vi "RunWireCalibration.vi"() -> ()   [LabVIEW 2016]
uses:
  Controls/0_XYZstage/BOOL_Moving.ctl
  <vilib>/userdefined/High Color/IMAQdx.ctl
  <vilib>/Utility/miscctls.llb/LVRowAndColumnUnsignedTypeDef.ctl
  <vilib>/Analysis/6fits.llb/Curve Fitting Criteria.ctl
  <extravilib>/ChannelInstances/High Speed Stream-c(i32,str,c(dbl,dbl),t'IMAQ Image.ctl',t'IMAQdx.ctl')/_Read For Replicate.vi
  Miscellaneous/PixelToMicron.vi
  <extravilib>/ChannelInstances/High Speed Stream-c(i32,str,c(dbl,dbl),t'IMAQ Image.ctl',t'IMAQdx.ctl')/Instantiate.vi
  <extravilib>/ChannelInstances/High Speed Stream-c(i32,str,c(dbl,dbl),t'IMAQ Image.ctl',t'IMAQdx.ctl')/)Channel.vi
  <extravilib>/ChannelInstances/High Speed Stream-c(i32,str,c(dbl,dbl),t'IMAQ Image.ctl',t'IMAQdx.ctl')/Abort Signal/Init Signal.vi
  <vilib>/gmath/statdist.llb/st_Percentiles (scalar).vi
  <vilib>/vision/driver/NI_Vision_Acquisition_Software.lvlib
  <vilib>/Analysis/NI_AALPro.lvlib
  <vilib>/Analysis/NI_AALBase.lvlib
  <vilib>/gmath/NI_Gmath.lvlib
  <vilib>/LabVIEW Interface for Arduino/LabVIEW Interface for Arduino.lvlib
  <extravilib>/ChannelInstances/High Speed Stream-c(i32,str,c(dbl,dbl),t'IMAQ Image.ctl',t'IMAQdx.ctl').lvlib
panel:
  out "completed":bool
  out "Loops":i32
  out "Image Data":T1(array[cluster])
  in  "Mode":enum16{"Run Calibration", "View Results"}(ring)
  out "Finished":bool
  in  "Tab Control":T2(tab)
  in  "error tab":bool
  in  "cam session":T3="cam1" caption="Select Camera"
  in  "Short-distance\naxis speed":T4={"vX [mm/s]"=5.0, "vY [mm/s]"=5.0, "vZ [mm/s]"=5.0}
  in  "Long-distance\naxis speed":T4={"vX [mm/s]"=25.0, "vY [mm/s]"=12.5, "vZ [mm/s]"=5.0}
  in  "wait time":u32=2000 caption="wait (ms)"
  in  "Y position":dbl=86.5 format="%#_13g"
  in  "Z position":dbl=30.25 format="%#_13g"
  in  "percentile":dbl=95.0 caption="tolerance percentile" format="%#_13g"
  in  "Python":path=path "python"
  in  "Wire Diameter":dbl=90.0 caption="Wire Diameter (microns)"
  in  "Image Info Results Read":path caption="Image Info Path"
  in  "Image File Results Read":bool=TRUE caption="View Images from Saved Location?"
  in  "Im. Source":T5(radio)
  out "Image Source Tab":T5(tab) caption="Warning: if you don't save the images, a new set of images must be captured to run the calibration again. Saving images allows the user to run the calibration on the same image set multiple times."
  in  "Save Images":bool=TRUE caption="Save Images to File?"
  in  "Image Calibration Write":path=path "C:/Users/Aerotech/Desktop/Joel Images 8_7" caption="Image Path"
  in  "Image Overwrite":bool=TRUE caption="Overwrite existing files?"
  in  "Image Info Calibration Read":path caption="Image Info Path"
  in  "View Results":bool
  in  "Data File Read":path caption="Data File Path"
  in  "Run Calibration":bool
  in  "File Name":string="data_file.csv"
  in  "Data File Overwrite":bool caption="Overwrite existing files?"
  in  "Data File Write":path=path "C:/Users/Aerotech/Desktop" caption="Data File Path"
  in  "List of All Fits":i32(listbox)
  out "Progress":dbl(slide) caption="Progress: 378/719" scale=0.0..100.0
  out "Moving":T6
  in  "abort":bool
  in  "pause":bool
  out "Graph of Fit":cluster{dbl[], dbl[]}[](graph) caption="Graph of Fit for Image #15"
  in  "List of Failed Fits":i32(listbox)
  out "Image":T7(plugin-control) caption="Image #15"
  out "Fit Info":T8={"Initial Guess"={"Center (pixels)"=-1.0, "Reflectivity"=0.0}, "Params Vector"=[], "Errors"=[], "Iterations"=0, "Success"=FALSE} {"Errors" format="%#_2g"; "Params Vector" format="%#_10f"; "Initial Guess"."Center (pixels)" format="%#_16g"}
  in  "Quit":bool
  out "Re-do Necessary?":bool
  out "fails":i32 caption="Number of Failed Fits:"
  out "Tolerance":dbl=4.0 caption="95% Tolerance (microns):" format="%_2g"
  out "Confidence":dbl caption="95% Confidence Interval (microns):" format="%.5g"
  out "std. dev.":dbl caption="Standard Deviation (microns):" format="%.5g"
  out "outside tolerance":bool caption="Within Tolerance?"
  out "Histogram of Final Fit Residuals":T9(graph) caption="XY Graph"
  out "Adjusted Graph of Final Fit":cluster{dbl[], dbl[]}(graph) caption="XY Graph"
  out "queue error":errorcluster
  out "image file error":errorcluster
  out "info file error":errorcluster
  out "Image Display Error":errorcluster
  out "data file write error":errorcluster
  out "Capture Error":errorcluster caption="stage/camera error"
  # "NOTE: Click \"RUN\" to run the VI BEFORE entering the set-up parameters!!!"
  # "For runnung a new calibration"
  # "For viewing a previously run calibration"
  # "Image Files"
  # "Settings"
  # "Image Files"
  # "Data File"
  # "Data File"
  # "Center (px)"
  # "Reflectivity (ul)"
  # "Amplitude (px val^2)"
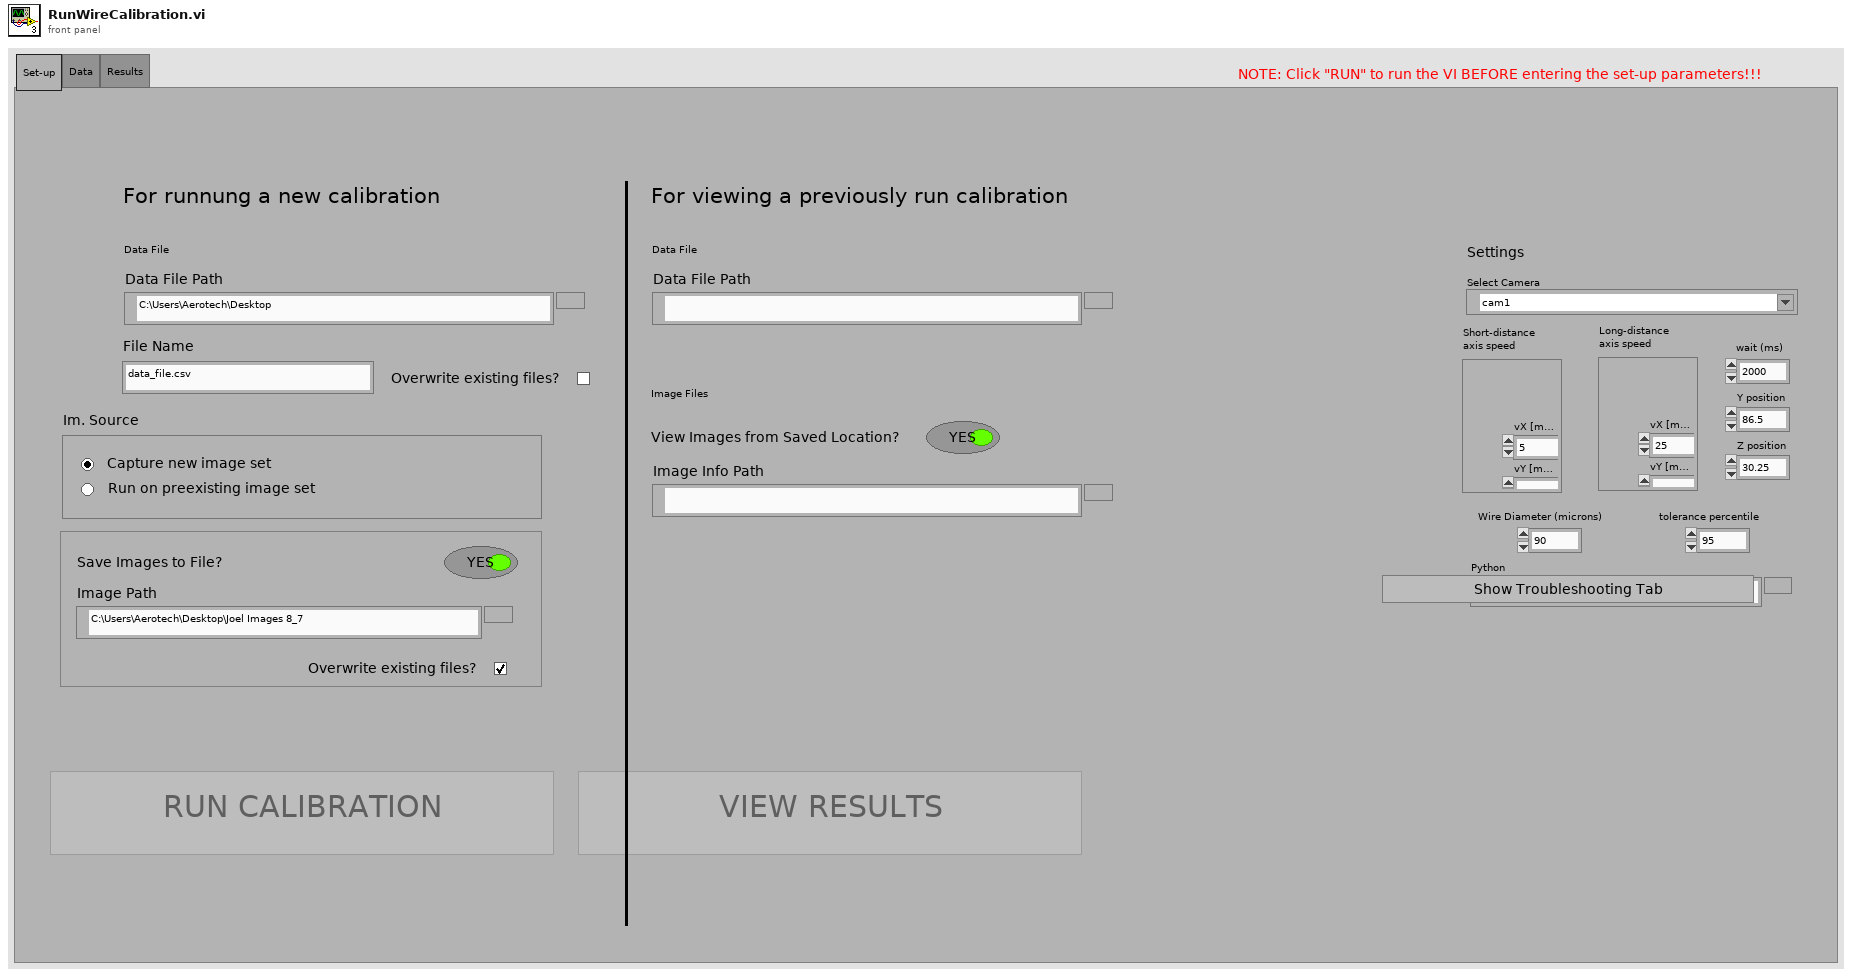
[diagram p1: front panel]
types:
  T1 = cluster{"success?":bool, "image number":i32, "camera position":cluster{"X":dbl, "Y":dbl}, "parameters":cluster{"amplitude":dbl, "center":dbl, "reflectivity":dbl}, "errors":cluster{"amplitude":dbl, "center":dbl, "reflectivity":dbl}, "Initial Guess":cluster{"center":dbl, "reflectivity":dbl}, "iterations":i32, "image path":path}[]
  T2 = enum32{"Set-up", "Data", "Results", "Troubleshooting"}
  T3 = typedef "IMAQdx.ctl" = refnum<k21>
  T4 = cluster{"vX [mm/s]":dbl, "vY [mm/s]":dbl, "vZ [mm/s]":dbl}
  T5 = enum32{"Capture new image set", "Run on preexisting image set"}
  T6 = typedef "BOOL_Moving.ctl" = bool
  T7 = typedef "IMAQ Image.ctl" = refnum<image>
  T8 = cluster{"Initial Guess":cluster{"Center (pixels)":dbl, "Reflectivity":dbl}, "Params Vector":dbl[], "Errors":dbl[], "Iterations":i32, "Success":bool}
  T9 = cluster{"X Values":dbl[], "Histogram: h(x)":i32[]}
  T10 = enum8{"Enabled", "Disabled", "Disabled and Grayed Out"}
  T11 = cluster{"Params Vector[1]":dbl, "Params Vector[2]":dbl}
  T12 = enum16{"open", "replace", "create", "open or create", "replace or create", "replace or create with confirmation"}
  T13 = cluster{"image number":i32, "image path":path, "position":cluster{dbl, dbl}}
  T14 = typedef "LVRowAndColumnUnsignedTypeDef.ctl" = cluster{"Row":u32, "Column":u32}
  T15 = cluster{"Data File Write":path, "File Name":string, "Data File Overwrite":bool}
  T16 = typedef "LabVIEW Interface for Arduino.lvlib/Arduino Resource.ctl" = cluster{"VISA resource":refnum<visa-resource-name>, "Board Type":T17, "Connection Type":enum8{"USB / Serial"}, "Bytes Per Packet (15)":u8}
  T17 = typedef "LabVIEW Interface for Arduino.lvlib/Board Type.ctl" = enum16{"Uno", "Dimuelanove w/Atmega 328", "Mega 2560"}
  T18 = typedef "ArduinoLT-ConfigurationControl.ctl" = cluster{"Lights: Digital I/O Pins":cluster{"Coaxial":u8, "Spotlights":u8}, "Thermistor Settings":cluster{"Analogue Readout Pin":u8, "Vcc Reference Pin":u8, "Paired Resistance (10K Ohms)":dbl, "Units (C)":enum16{"Celsius", "Fahrenheit", "Kelvin"}}}
  T19 = cluster{"Image Calibration Write":path, "Image Overwrite":bool}
  T20 = cluster{"Arduino Configuration OUT":T18, "Arduino Resource OUT":T16, "error out":errorcluster}
  T21 = typedef "Image Type" = u32
  T22 = cluster{"Final X":dbl, "Final Y":dbl, "Final Z":dbl}
  T23 = cluster{i32, string, cluster{"Final X":dbl, "Final Y":dbl}, "Image Out":T7, "Session Out":T3}
  T24 = typedef "High Speed Stream-c(i32,str,c(dbl,dbl),t'IMAQ Image.ctl',t'IMAQdx.ctl').lvlib/)Channel.ctl" = refnum<queue>
  T25 = cluster{i32, "Smart Path":path, cluster{"Final X":dbl, "Final Y":dbl}}
  T26 = cluster{i32, "appended path":path, cluster{dbl, dbl}}
  T27 = cluster{"Params Vector[0]":dbl, "Params Vector[1]":dbl, "Params Vector[2]":dbl}
  T28 = cluster{"Errors[0]":dbl, "Errors[1]":dbl, "Errors[2]":dbl}
  T29 = cluster{"Success":bool, "image number":i32, "position":cluster{dbl, dbl}, "Params Vector":cluster{"Params Vector[0]":dbl, "Params Vector[1]":dbl, "Params Vector[2]":dbl}, "Errors":cluster{"Errors[0]":dbl, "Errors[1]":dbl, "Errors[2]":dbl}, cluster{"Params Vector[1]":dbl, "Params Vector[2]":dbl}, "Iterations":i32, "image path":path}
  T30 = cluster{"Success":bool, "image number":i32, "position":cluster{"X":dbl, "Y":dbl}, "Params Vector":cluster{"Params Vector[0]":dbl, "Params Vector[1]":dbl, "Params Vector[2]":dbl}, "Errors":cluster{"Errors[0]":dbl, "Errors[1]":dbl, "Errors[2]":dbl}, "Initial Guess":cluster{"Params Vector[1]":dbl, "Params Vector[2]":dbl}, "Iterations":i32, "image path":path}[]
  T31 = cluster{bool, i32, cluster{dbl, dbl}, cluster{dbl, dbl, dbl}, cluster{dbl, dbl, dbl}, cluster{dbl, dbl}, i32, "appended path":path}
  T32 = typedef "NI_AALPro.lvlib/Curve Fitting Criteria.ctl" = u16
  T33 = cluster{"success?":bool, "image number":i32, "camera position":cluster{"X":dbl, "Y":dbl}, "parameters":cluster{"amplitude":dbl, "center":dbl, "reflectivity":dbl}, "errors":cluster{"amplitude":dbl, "center":dbl, "reflectivity":dbl}, "Initial Guess":cluster{"center":dbl, "reflectivity":dbl}, "iterations":i32, "image path":path}
  T34 = cluster{"amplitude":dbl, "center":dbl, "reflectivity":dbl}
  T35 = cluster{"Initial Guess":cluster{"center":dbl, "reflectivity":dbl}, "parameters":dbl[], "errors":dbl[], "iterations":i32, "success?":bool}
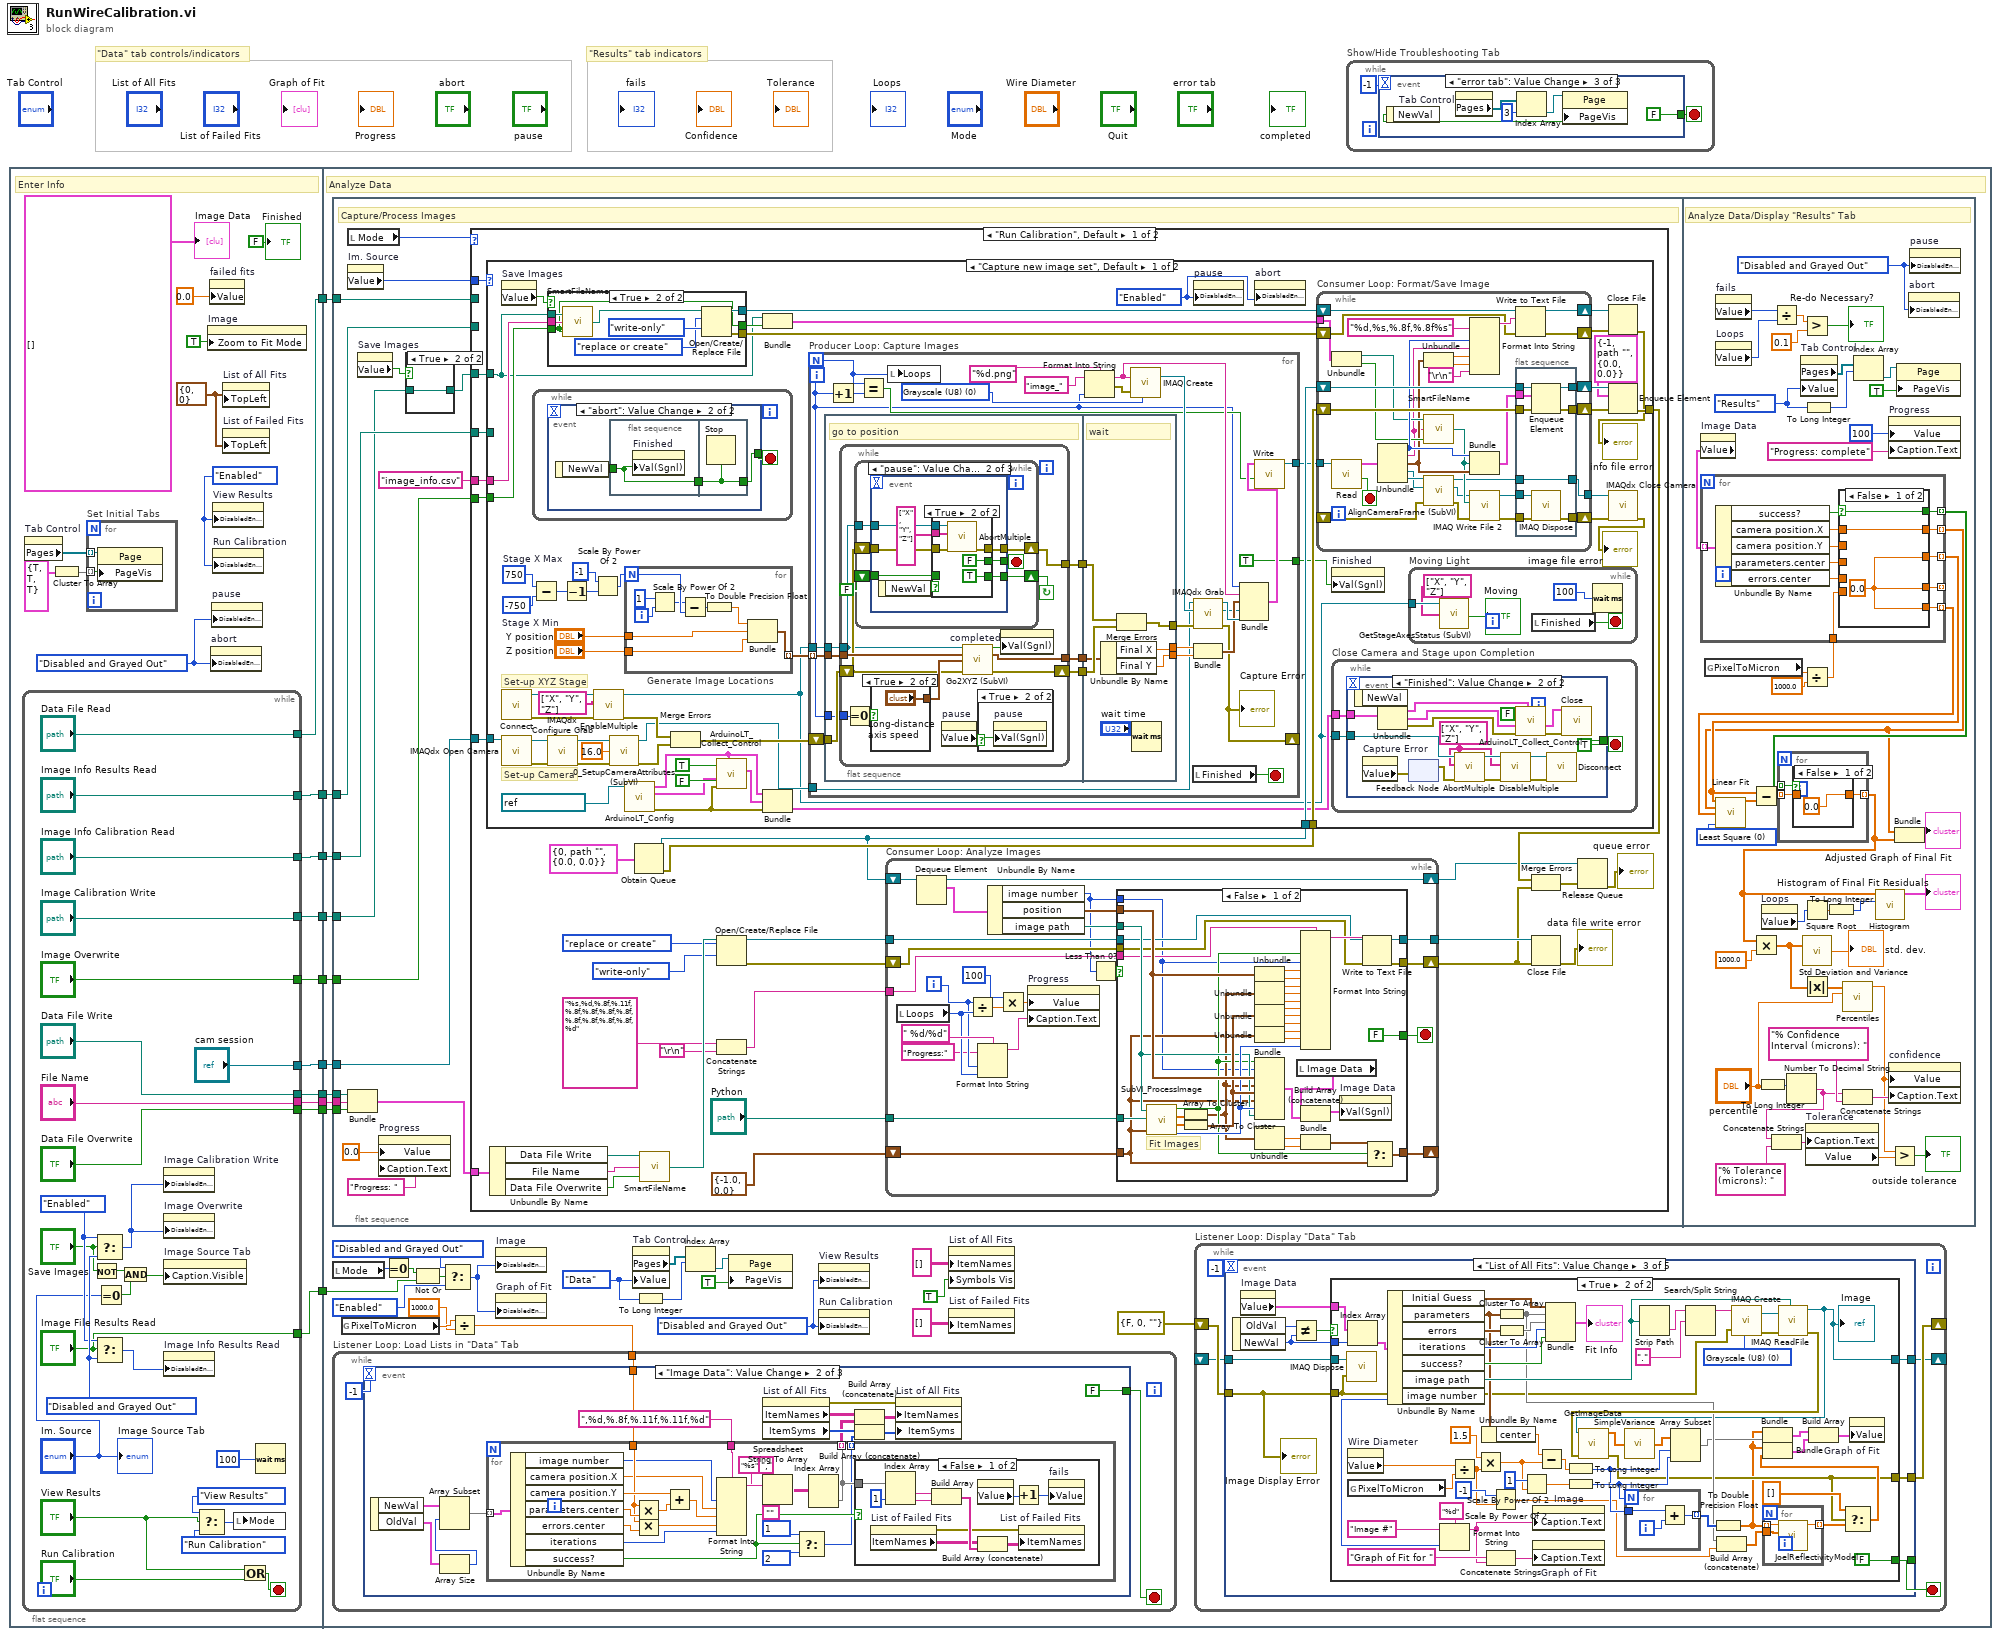
[diagram p0: block diagram]
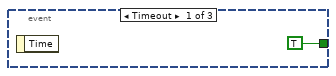
[diagram p2: hidden frame]
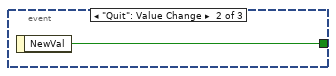
[diagram p3: hidden frame]
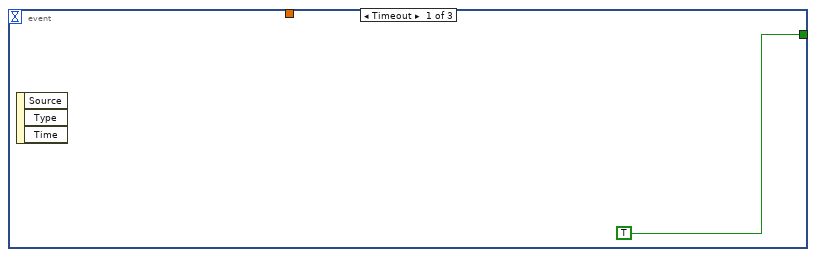
[diagram p4: hidden frame]
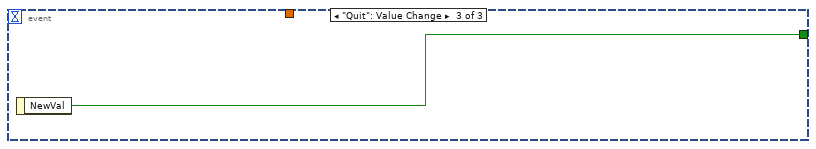
[diagram p6: hidden frame]
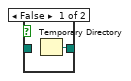
[diagram p7: hidden frame]
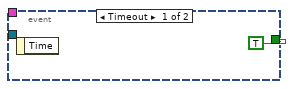
[diagram p8: hidden frame]
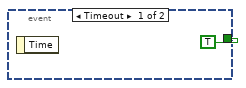
[diagram p9: hidden frame]
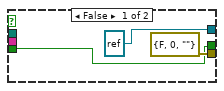
[diagram p10: hidden frame]
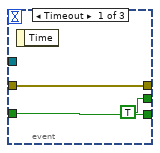
[diagram p12: hidden frame]
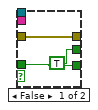
[diagram p13: hidden frame]
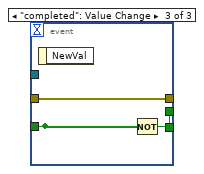
[diagram p14: hidden frame]
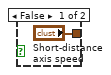
[diagram p15: hidden frame]
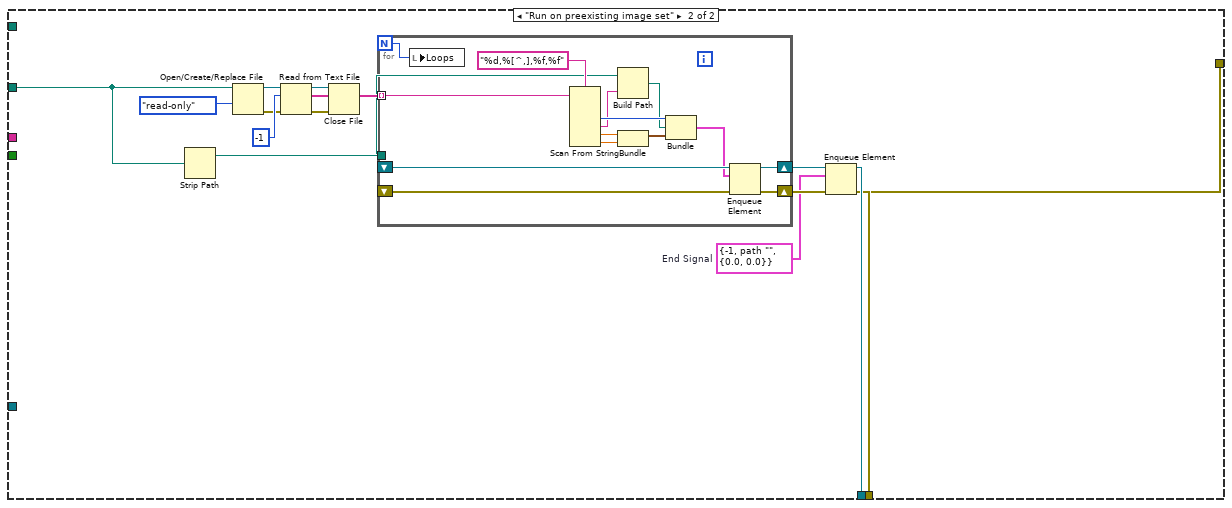
[diagram p16: hidden frame]
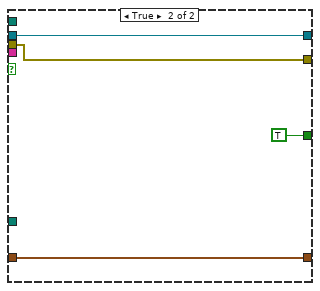
[diagram p17: hidden frame]
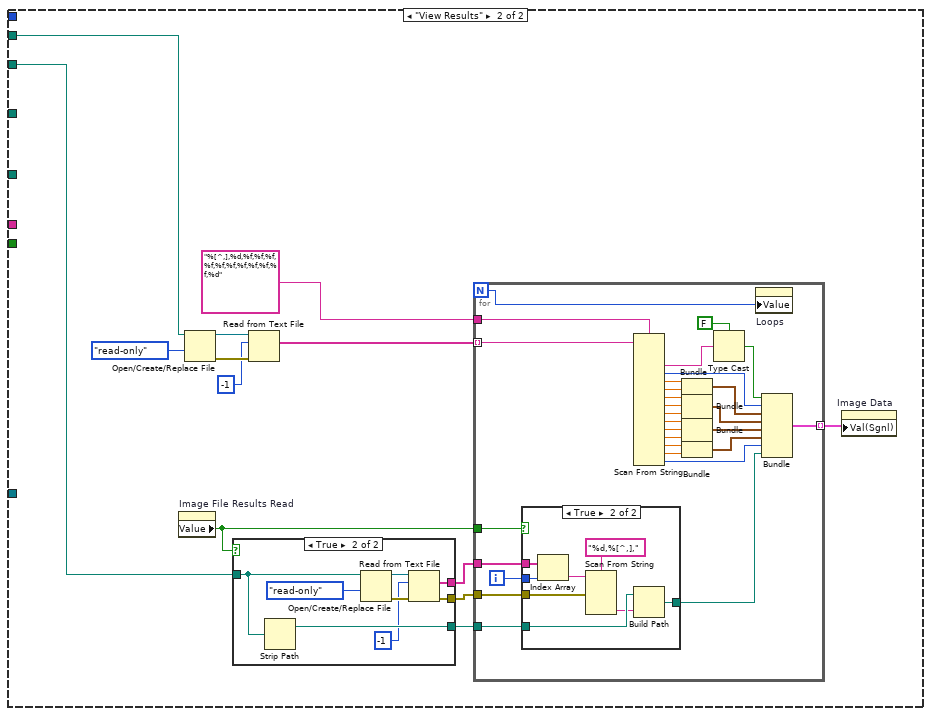
[diagram p18: hidden frame]
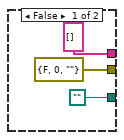
[diagram p19: hidden frame]
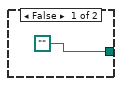
[diagram p20: hidden frame]
diagram:
  # "\"Results\" tab indicators"
  # "\"Data\" tab controls/indicators"
  n1 = flat-sequence {
    tunnel: [w21] -> w10
    tunnel: [w23] -> w9
    tunnel: [w29] -> w8
    tunnel: [w28] -> w7
    tunnel: [w27] -> w6
    tunnel: [w26] -> w5
    tunnel: [w25] -> w4
    tunnel: [w24] -> w3
    tunnel: [w22] -> w2
    tunnel: [w14] -> w1
    tunnel: w10 -> [w79]
    tunnel: w9 -> [w78]
    tunnel: w8 -> [w77]
    tunnel: w7 -> [w72]
    tunnel: w6 -> [w71]
    tunnel: w5 -> [w70]
    tunnel: w4 -> [w69]
    tunnel: w3 -> [w68]
    tunnel: w2 -> [w67]
    tunnel: w1 -> [w60]
    frame #0 {
      w12 = T10."Disabled and Grayed Out" ("Disabled")
      w13 = T10."Enabled" ("Disabled")
      w18 = T14 {"Row"=0, "Column"=0} ("Top Left Visible Cell")
      # "Enter Info"
      n2 = while {
        tunnel: ["Image Overwrite"] -> w29
        tunnel: ["Data File Write"] -> w28
        tunnel: ["File Name"] -> w27
        tunnel: ["Data File Overwrite"] -> w26
        tunnel: ["cam session"] -> w25
        tunnel: ["Image Calibration Write"] -> w24
        tunnel: ["Image Info Calibration Read"] -> w23
        tunnel: ["Image Info Results Read"] -> w22
        tunnel: ["Data File Read"] -> w21
        tunnel: ["Image File Results Read"] -> w14
        stop <- w46 stop-if-true
        w53 = T10."Enabled" ("Disabled")
        w54 = T10."Disabled and Grayed Out" ("Disabled")
        n3 = Not(x="Save Images") -> (.not. x?=w38:bool)
        n4 = Select(t=w53, s="Save Images", f=w54) -> (s? t:f=w52:T10)
        n5 = Select(t=w53, s="Image File Results Read", f=w54) -> (s? t:f=w40:T10)
        n6 = Equal To 0?(x="Im. Source") -> (x = 0?=w36:bool)
        n7 = And(x=w38, y=w36) -> (x .and. y?=w37:bool)
        n8 = property on="Image Calibration Write" class="Path"("DisabledEnum"=w52) -> ()  [unwired: 2 in, 2 out]
        n9 = property on="Image Overwrite" class="Bool (strict)"("DisabledEnum"=w52) -> ()  [unwired: 2 in, 2 out]
        n10 = property on="Image Source Tab" class="TabCtl (strict)"("Caption.Visible"=w37) -> ()  [unwired: 2 in, 2 out]
        n11 = property on="Image Info Results Read" class="Path"("DisabledEnum"=w40) -> ()  [unwired: 2 in, 2 out]
        n12 = Select(t=enum16{"Run Calibration", "View Results"}."View Results" ("Mode"), s="View Results", f=enum16{"Run Calibration", "View Results"}."Run Calibration" ("Mode")) -> (s? t:f=w51:enum16{"Run Calibration", "View Results"})
        n13 = local write "Mode"(w51) -> ()
        n14 = Or(x="View Results", y="Run Calibration") -> (x .or. y?=w46:bool)
        n15 = Wait (ms)(milliseconds to wait=u32 100) -> ()  [unwired: 1 out]
        "Image Source Tab" <- "Im. Source"
      }
      n16 = property on="Tab Control" class="TabCtl (strict)"() -> ("Pages"=w17:refnum<vi>[])  [unwired: 2 in, 2 out]
      n17 = Cluster To Array(cluster=cluster{bool, bool, bool} {TRUE, TRUE, TRUE}) -> (array=w15:bool[])
      n18 = for "Set Initial Tabs" {
        tunnel: w17 -> [w32] mode=indexing
        tunnel: w15 -> [w31] mode=indexing
        n19 = property class="Page"(reference=w32, "PageVis"=w31) -> ()  [unwired: 1 in, 2 out]
      }
      n20 = property on="Image" class="ImageControl"("Zoom to Fit Mode"=TRUE) -> ()  [unwired: 2 in, 2 out]
      n21 = property on="failed fits" class="DigNum (strict)"("Value"=0.0 ("Number of Failed Fits:")) -> ()  [unwired: 2 in, 2 out]
      n22 = property on="abort" class="Bool"("DisabledEnum"=w12) -> ()  [unwired: 2 in, 2 out]
      n23 = property on="pause" class="Bool (strict)"("DisabledEnum"=w12) -> ()  [unwired: 2 in, 2 out]
      n24 = property on="View Results" class="Bool"("DisabledEnum"=w13) -> ()  [unwired: 2 in, 2 out]
      n25 = property on="Run Calibration" class="Bool"("DisabledEnum"=w13) -> ()  [unwired: 2 in, 2 out]
      n26 = property on="List of All Fits" class="MCListbox (strict)"("TopLeft"=w18) -> ()  [unwired: 2 in, 2 out]
      n27 = property on="List of Failed Fits" class="MCListbox (strict)"("TopLeft"=w18) -> ()  [unwired: 2 in, 2 out]
      "Image Data" <- T1 []
      "Finished" <- FALSE ("Finished")
    }
    frame #1 {
      w59 = T10."Disabled and Grayed Out" ("Disabled")
      w81 = T2."Data" ("Tab Control")
      # "Analyze Data"
      n28 = flat-sequence {
        tunnel: w79 -> [w153]
        tunnel: w78 -> [w142]
        tunnel: w77 -> [w152]
        tunnel: w72 -> [w150]
        tunnel: w71 -> [w149]
        tunnel: w70 -> [w148]
        tunnel: w69 -> [w146]
        tunnel: w68 -> [w140]
        tunnel: w67 -> [w145]
        frame #0 {
          # "Capture/Process Images"
          n29 = local read "Mode"() -> (w155:enum16{"Run Calibration", "View Results"})
          n30 = property on="Im. Source" class="RadioBtnsControl (strict)"() -> ("Value"=w154:T5)  [unwired: 2 in, 2 out]
          n31 = Bundle("Data File Write"=w150, "File Name"=w149, "Data File Overwrite"=w148) -> (w147:T15)  [unwired: 1 in]
          n32 = property on="Save Images" class="Bool (strict)"() -> ("Value"=w139:bool)  [unwired: 2 in, 2 out]
          n33 = property on="Progress" class="Slide (strict)"("Value"=0.0 ("Progress"), "Caption.Text"="Progress: ") -> ()  [unwired: 2 in, 2 out]
          n34 = case shown="True" w139 {
            tunnel: [w156 w157] -> w141
            tunnel: w140 -> [_ w157]
            frame False {
              n35 = Temporary Directory() -> (w156:path)
            }
            frame True {
            }
          }
          n36 = case shown="\"Run Calibration\", Default" w155 {
            tunnel: w154 -> [w186 _]
            tunnel: w147 -> [w180 _]
            tunnel: w153 -> [_ w529]
            tunnel: w145 -> [_ w523]
            tunnel: w142 -> [w179 _]
            tunnel: w146 -> [w178 _]
            tunnel: w152 -> [w177 _]
            tunnel: "image_info.csv" -> [w174 _]
            tunnel: w141 -> [w162 _]
            frame "Run Calibration", Default {
              n37 = Unbundle By Name(w180) -> ("Data File Write"=w160:path, "File Name"=w159:string, "Data File Overwrite"=w158:bool)
              n38 = Obtain Queue(element data type=T13 {"image number"=0, "image path"=path "", "position"={0.0, 0.0}} ("Cluster")) -> (queue out=w171:refnum<queue>, error out=w184:errorcluster)  [unwired: 4 in, 1 out]
              n39 = case shown="\"Capture new image set\", Default" w186 {
                tunnel: w184 -> [w208 w436]
                tunnel: w179 -> [_ w432]
                tunnel: w178 -> [w225 _]
                tunnel: w177 -> [w197 _]
                tunnel: w171 -> [w207 w437]
                tunnel: [w209 w426] -> w175
                tunnel: w174 -> [w195 _]
                tunnel: w162 -> [w189 _]
                frame "Capture new image set", Default {
                  w190 = T10."Enabled" ("Disabled")
                  w232 = 750  # Stage X Max
                  w231 = -750  # Stage X Min
                  # "Set-up XYZ Stage"
                  # "Set-up Camera"
                  n40 = property on="Save Images" class="Bool (strict)"() -> ("Value"=w216:bool)  [unwired: 2 in, 2 out]
                  n41 = call "Connect.vi"() -> ("error out"=w234:errorcluster, "controller"=w233:refnum<k24>)  [unwired: 10 in]
                  n42 = call <vilib>:"IMAQdx Open Camera.vi"("Session In"=w225) -> ("error out"=w239:errorcluster, "Session Out"=w240:T3)  [unwired: 2 in, 7 out]
                  n43 = Subtract(x=w232, y=w231) -> (x-y=w230:i32)
                  n44 = while {
                    stop <- w262 stop-if-true
                    n45 = event shown="[1] \"abort\": Value Change" {
                      selector: _ -> [_ _]
                      dyn-events: _ -> [_ _]
                      timeout: _ -> [_ _]
                      tunnel: [TRUE w264] -> w262
                      event Timeout {
                        n46 = event-data() -> ()  [unwired: 1 in, 1 out]
                      }
                      event "abort": Value Change {
                        n47 = event-data() -> ("NewVal"=w266:bool)  [unwired: 1 in]
                        n48 = flat-sequence {
                          tunnel: w266 -> [w267]
                          tunnel: [w267] -> w265
                          tunnel: w265 -> [w268]
                          tunnel: [w268] -> w264
                          frame #0 {
                            n49 = property on="Finished" class="Bool (strict)"("Val(Sgnl)"=w267) -> ()  [unwired: 2 in, 2 out]
                          }
                          frame #1 {
                            n50 = Stop(stop? (T)=w268) -> ()
                          }
                        }
                      }
                    }
                  }
                  n51 = case shown="True" w216 {
                    tunnel: w197 -> [w317 w321]
                    tunnel: [refnum<file> refnum ("refnum out") w326] -> w206
                    tunnel: [errorcluster {"status"=FALSE, "code"=0, "source"=""} ("error out") w325] -> w205
                    tunnel: w189 -> [_ w323]
                    tunnel: [w317 w321] -> w196
                    tunnel: w195 -> [_ w322]
                    frame False {
                    }
                    frame True {
                      n52 = call "SmartFileName.vi"("Allow Replacement (False)"=w321, "preferred name"=w322, "preferred path"=w323) -> ("Smart Path"=w320:path)
                      n53 = Open/Create/Replace File(file path (use dialog)=w320, operation (0:open)=T12."replace or create", access (0:read/write)=enum16{"read/write", "read-only", "write-only"}."write-only") -> (refnum out=w326:refnum<file>, error out=w325:errorcluster)  [unwired: 3 in, 1 out]
                    }
                  }
                  n54 = call <vilib>:"IMAQdx Configure Grab.vi"("error in"=w239, "Session In"=w240) -> ("error out"=w237:errorcluster, "Session Out"=w238:T3)  [unwired: 8 out]
                  n55 = Decrement(x=w230) -> (x-1=w229:i32)
                  n56 = Scale By Power Of 2(n=i8 -1, x=w229) -> (x*2^n=w227:i32)
                  n57 = call "EnableMultiple.vi"("error in (no error)"=w234, "axis names"=string[] ["X", "Y", "Z"], "controller in"=w233) -> ("error out"=w224:errorcluster, "controller out"=w192:refnum<k24>)  [unwired: 7 in]
                  n58 = call "0_SetupCameraAttributes (SubVI).vi"("error in (no error)"=w237, "Gain"=16.0, "Camera session in"=w238) -> ("error out"=w223:errorcluster, "Camera session out"=w204:T3)  [unwired: 7 in]
                  n59 = for "Generate Image Locations" {
                    N: w227 -> [w421]
                    tunnel: [w418] -> w226 mode=indexing
                    tunnel: "Y position" -> [w416]
                    tunnel: "Z position" -> [w415]
                    i -> [w423]
                    n60 = Scale By Power Of 2(n=i8 1, x=w423) -> (x*2^n=w420:i32)
                    n61 = Subtract(x=w420, y=w421) -> (x-y=w419:i32)
                    n62 = To Double Precision Float(number=w419) -> (double precision float=w417:dbl)
                    n63 = Bundle(w417, "Y position"=w416, "Z position"=w415) -> (w418:cluster{dbl, "Y position":dbl, "Z position":dbl})  [unwired: 1 in]
                  }
                  n64 = call "ArduinoLT_Config.vi"("VISA resource"=refnum<visa-resource-name> "LightsCTRL") -> ("error out"=w199:errorcluster, "Arduino Resource"=w217:T16, "Arduino Configuration OUT"=w188:T18)  [unwired: 4 in, 1 out]
                  n65 = Merge Errors(w224, w223) -> (w222:errorcluster)
                  n66 = call "ArduinoLT_Collect_Control.vi"("Arduino Configuration"=w188, "error in"=w199, "Arduino Resource IN"=w217, "Spotlights"=FALSE, "Coaxial light"=TRUE) -> ("Arduino Resource OUT"=w200:T16)  [unwired: 4 in, 2 out]
                  n67 = Bundle("Image Calibration Write"=w189, "Image Overwrite"=w196) -> (w203:T19)  [unwired: 1 in]
                  n68 = Bundle("Arduino Configuration OUT"=w188, "Arduino Resource OUT"=w200, "error out"=w199) -> (w193:T20)  [unwired: 1 in]
                  n69 = for "Producer Loop: Capture Images" {
                    N -> [w340]
                    tunnel: w204 -> [w331]
                    tunnel: w192 -> [w355]
                    tunnel: w226 -> [w345] mode=indexing
                    tunnel: [TRUE] -> w198
                    shift-right: [w329] -> _
                    shift-left: w222 -> [w354]
                    tunnel: [w335] -> w191
                    i -> [w330]
                    stop <- w334 stop-if-true
                    w350 = T21 0 items=["Grayscale (U8)", "Grayscale (I16)", "Grayscale (SGL)", "Complex (CSG)", "RGB (U32)", "HSL (U32)", "RGB (U64)", "Grayscale (U16)"] ("Image Type")
                    n70 = flat-sequence {
                      tunnel: w345 -> [w362]
                      tunnel: w355 -> [w356]
                      tunnel: w354 -> [w361]
                      tunnel: [w360] -> w353
                      tunnel: [w359] -> w344
                      tunnel: [w358] -> w332
                      tunnel: w330 -> [w357]
                      tunnel: w353 -> [w413]
                      tunnel: [w409] -> w352
                      tunnel: w344 -> [w412]
                      tunnel: [w411] -> w343
                      tunnel: [w410] -> w342
                      tunnel: w332 -> [w408]
                      frame #0 {
                        # "go to position"
                        n71 = while {
                          shift-right: [w374] -> w360
                          shift-left: w361 -> [w369]
                          tunnel: w362 -> [w375]
                          tunnel: [w372] -> w359
                          tunnel: [w368] -> w358
                          tunnel: w357 -> [w366]
                          tunnel: w356 -> [w365]
                          stop <- w370 continue-if-true
                          n72 = Equal To 0?(x=w366) -> (x = 0?=w367:bool)
                          n73 = while {
                            shift-right: [w382] -> w368
                            shift-left: w369 -> [w381]
                            shift-right: [w380] -> w370
                            shift-left: FALSE -> [w379]
                            tunnel: w365 -> [w377]
                            stop <- w378 stop-if-true
                            n74 = event shown="[1] \"pause\": Value Change" {
                              selector: _ -> [_ _ _]
                              dyn-events: _ -> [_ _ _]
                              timeout: _ -> [_ _ _]
                              tunnel: [w385 w393 w405] -> w382
                              tunnel: w381 -> [w385 w392 w405]
                              tunnel: [w384 w390 w403] -> w380
                              tunnel: w379 -> [w384 w389 w403]
                              tunnel: [TRUE ("NewVal") w388 w404] -> w378
                              tunnel: w377 -> [_ w386 _]
                              event Timeout {
                                n75 = event-data() -> ()  [unwired: 1 in, 1 out]
                              }
                              event "pause": Value Change {
                                n76 = event-data() -> ("NewVal"=w391:bool)  [unwired: 1 in]
                                n77 = case shown="True" w391 {
                                tunnel: [w395 w402] -> w393
                                tunnel: string[] ["X", "Y", "Z"] ("axis names") -> [_ w401]
                                tunnel: w392 -> [w395 w400]
                                tunnel: [w396 TRUE] -> w390
                                tunnel: w389 -> [w396 _]
                                tunnel: [TRUE ("NewVal") FALSE ("NewVal")] -> w388
                                tunnel: w386 -> [_ w397]
                                frame False {
                                }
                                frame True {
                                n78 = call "AbortMultiple.vi"("error in (no error)"=w400, "axis names"=w401, "controller in"=w397) -> ("error out"=w402:errorcluster)  [unwired: 7 in, 1 out]
                                }
                                }
                              }
                              event "completed": Value Change {
                                n79 = event-data() -> ()  [unwired: 1 in, 1 out]
                                n80 = Not(x=w403) -> (.not. x?=w404:bool)
                              }
                            }
                          }
                          n81 = case shown="True" w367 {
                            tunnel: ["Short-distance\naxis speed" "Long-distance\naxis speed"] -> w373
                            frame False {
                            }
                            frame True {
                            }
                          }
                          n82 = property on="pause" class="Bool (strict)"() -> ("Value"=w363:bool)  [unwired: 2 in, 2 out]
                          n83 = call "Go2XYZ (SubVI).vi"(".NET Refnum in"=w365, "Go to Coordinates"=w375, "Axis Speeds"=w373, "error in (no error)"=w369) -> ("completed"=w371:bool, "Final Position"=w372:T22, "error out"=w374:errorcluster)  [unwired: 7 in, 2 out]
                          n84 = case shown="True" w363 {
                            selector: w363 -> [_ w376]
                            frame False {
                            }
                            frame True {
                              n85 = property on="pause" class="Bool (strict)"("Val(Sgnl)"=w376) -> ()  [unwired: 2 in, 2 out]
                            }
                          }
                          n86 = property on="completed" class="Bool (strict)"("Val(Sgnl)"=w371) -> ()  [unwired: 2 in, 2 out]
                        }
                      }
                      frame #1 {
                        # "wait"
                        n87 = Unbundle By Name(w412) -> ("Final X"=w410:dbl, "Final Y"=w411:dbl)
                        n88 = Merge Errors(w408, w413) -> (w409:errorcluster)
                        n89 = Wait (ms)(milliseconds to wait="wait time") -> ()  [unwired: 1 out]
                      }
                    }
                    n90 = Increment(x=w330) -> (x+1=w341:i32)
                    n91 = Equal?(x=w340, y=w341) -> (x = y?=w336:bool)
                    n92 = local write "Loops"(w340) -> ()
                    n93 = Format Into String(format string="%d.png", initial string="image_", w330) -> (resulting string=w346:string, error out=w349:errorcluster)  [unwired: 1 in]
                    n94 = call "IMAQ Create"("Image Name"=w346, "Image Type"=w350, "error in (no error)"=w349) -> ("New Image"=w348:T7)  [unwired: 1 in, 2 out]
                    n95 = local read "Finished"() -> (w334:bool)
                    n96 = call <vilib>:"IMAQdx Grab.vi"("error in"=w352, "Image In"=w348, "Session In"=w331) -> ("error out"=w329:errorcluster, "Image Out"=w328:T7, "Session Out"=w339:T3)  [unwired: 1 in, 5 out]
                    "Capture Error" <- w329
                    n97 = Bundle("Final X"=w342, "Final Y"=w343) -> (w338:cluster{"Final X":dbl, "Final Y":dbl})  [unwired: 1 in]
                    n98 = Bundle(w330, w346, w338, "Image Out"=w328, "Session Out"=w339) -> (w337:T23)  [unwired: 1 in]
                    n99 = call <extravilib>:"Write.vi"("last element? (F)"=w336, "element"=w337) -> ("channel"=w335:T24)  [unwired: 7 in, 2 out]
                  }
                  n100 = property on="pause" class="Bool (strict)"("DisabledEnum"=w190) -> ()  [unwired: 2 in, 2 out]
                  n101 = property on="abort" class="Bool"("DisabledEnum"=w190) -> ()  [unwired: 2 in, 2 out]
                  n102 = while "Consumer Loop: Format/Save Image" {
                    tunnel: w191 -> [w276]
                    shift-right: [w298] -> w213
                    shift-left: w208 -> [w297]
                    shift-right: [w288] -> w215
                    shift-left: w205 -> [w289]
                    shift-right: [w287] -> w212
                    shift-left: w207 -> [w299]
                    shift-right: [w286] -> w214
                    shift-left: w206 -> [w290]
                    shift-right: [w300] -> w210
                    shift-left: _ -> [w283]
                    tunnel: w203 -> [w280]
                    tunnel: [w269] -> w202
                    stop <- w275 stop-if-true
                    n103 = Unbundle(w280) -> ("Image Calibration Write"=w281:path, "Image Overwrite"=w282:bool)
                    n104 = call <extravilib>:"Read.vi"("channel"=w276) -> ("done?"=w275:bool, "element"=w274:T23)  [unwired: 6 in, 3 out]
                    n105 = Unbundle(w274) -> (w295:i32, w271:string, w277:cluster{"Final X":dbl, "Final Y":dbl}, "Image Out"=w278:T7, "Session Out"=w279:T3)
                    n106 = Unbundle(w277) -> ("Final X"=w294:dbl, "Final Y"=w293:dbl)
                    n107 = call "SmartFileName.vi"("Allow Replacement (False)"=w282, "preferred name"=w271, "preferred path"=w281) -> ("Smart Path"=w273:path)
                    n108 = call "AlignCameraFrame (SubVI).vi"("error in (no error)"=w283, "Image Src"=w278, "Camera session in"=w279) -> ("error out"=w284:errorcluster, "Image Dst Out"=w272:T7, "Camera session out"=w270:T3)  [unwired: 6 in]
                    n109 = Format Into String(format string="%d,%s,%.8f,%.8f%s", w295, w271, w294, w293, "\r\n") -> (resulting string=w291:string)  [unwired: 2 in, 1 out]
                    n110 = Bundle(w295, "Smart Path"=w273, w277) -> (w296:T25)  [unwired: 1 in]
                    n111 = call-poly "IMAQ Write File 2"("error in (no error)"=w284, "File Path"=w273, "Image"=w272) -> ("error out"=w302:errorcluster, "Image Out (duplicate)"=w301:T7)  [unwired: 7 in]
                    n112 = Write to Text File(file (use dialog)=w290, text=w291, error in=w289) -> (refnum out=w286:refnum<file>, error out=w288:errorcluster)  [unwired: 1 in, 1 out]
                    n113 = flat-sequence {
                      tunnel: w302 -> [w311]
                      tunnel: w301 -> [w310]
                      tunnel: [w309] -> w300
                      tunnel: w299 -> [w308]
                      tunnel: [w307] -> w298
                      tunnel: w297 -> [w306]
                      tunnel: w296 -> [w305]
                      tunnel: [w304] -> w287
                      tunnel: w270 -> [w303]
                      tunnel: [w303] -> w269
                      frame #0 {
                        n114 = Enqueue Element(queue=w308, element=w305, error in (no error)=w306) -> (queue out=w304:refnum<queue>, error out=w307:errorcluster)  [unwired: 1 in, 1 out]
                        n115 = call "IMAQ Dispose"("Image"=w310, "error in (no error)"=w311) -> ("error out"=w309:errorcluster)  [unwired: 4 in]
                      }
                    }
                  }
                  n116 = property on="Finished" class="Bool (strict)"("Val(Sgnl)"=w198) -> ()  [unwired: 2 in, 2 out]
                  n117 = while "Close Camera and Stage upon Completion" {
                    tunnel: w193 -> [w243]
                    tunnel: w192 -> [w242]
                    stop <- w244 stop-if-true
                    n118 = event shown="[1] \"Finished\": Value Change" {
                      selector: _ -> [_ _]
                      dyn-events: _ -> [_ _]
                      timeout: _ -> [_ _]
                      tunnel: [TRUE TRUE] -> w244
                      tunnel: w243 -> [_ w258]
                      tunnel: w242 -> [_ w257]
                      event Timeout {
                        n119 = event-data() -> ()  [unwired: 1 in, 1 out]
                      }
                      event "Finished": Value Change {
                        w249 = FALSE ("Spotlights")
                        w255 = string[] ["X", "Y", "Z"] ("axis names")
                        n120 = event-data() -> ()  [unwired: 1 in, 1 out]
                        n121 = property on="Capture Error" class="Clust (strict)"() -> ("Value"=w253:errorcluster)  [unwired: 2 in, 2 out]
                        n122 = Unbundle(w258) -> ("Arduino Configuration OUT"=w246:T18, "Arduino Resource OUT"=w247:T16, "error out"=w248:errorcluster)
                        n123 = feedback-in #1(w253) -> ()
                        n124 = feedback #1() -> (w252:errorcluster)  [unwired: 1 in]
                        n125 = call "AbortMultiple.vi"("error in (no error)"=w252, "axis names"=w255, "controller in"=w257) -> ("error out"=w254:errorcluster, "controller out"=w256:refnum<k24>)  [unwired: 7 in]
                        n126 = call "DisableMultiple.vi"("error in (no error)"=w254, "axis names"=w255, "controller in"=w256) -> ("error out"=w260:errorcluster, "controller out"=w261:refnum<k24>)  [unwired: 7 in]
                        n127 = call "ArduinoLT_Collect_Control.vi"("Arduino Configuration"=w246, "error in"=w248, "Arduino Resource IN"=w247, "Spotlights"=w249, "Coaxial light"=w249) -> ("error out"=w250:errorcluster, "Arduino Resource OUT"=w251:T16)  [unwired: 4 in, 1 out]
                        n128 = call "Disconnect.vi"("error in (no error)"=w260, "controller"=w261) -> ()  [unwired: 9 in, 1 out]
                        n129 = call <vilib>:"Close.vi"("Arduino Resource"=w251, "error in"=w250) -> ()  [unwired: 13 in, 1 out]
                      }
                    }
                  }
                  n130 = while "Moving Light" {
                    tunnel: w192 -> [w315]
                    stop <- w312 stop-if-true
                    n131 = call "GetStageAxesStatus (SubVI).vi"(".NET Refnum in - Device"=w315, "Axes Names"=string[] ["X", "Y", "Z"] ("axis names")) -> ("Moving"=→"Moving":bool)  [unwired: 1 in, 7 out]
                    n132 = local read "Finished"() -> (w312:bool)
                    n133 = Wait (ms)(milliseconds to wait=u32 100) -> ()  [unwired: 1 out]
                  }
                  n134 = Close File(refnum=w214, error in=w215) -> (error out=→"info file error":errorcluster)  [unwired: 1 out]
                  n135 = Enqueue Element(queue=w212, element=T13 {"image number"=-1, "image path"=path "", "position"={0.0, 0.0}} ("End Signal"), error in (no error)=w213) -> (error out=w209:errorcluster)  [unwired: 1 in, 2 out]
                  n136 = call <vilib>:"IMAQdx Close Camera.vi"("error in"=w210, "Session In"=w202) -> ("error out"=→"image file error":errorcluster)  [unwired: 9 out]
                }
                frame "Run on preexisting image set" {
                  w424 = T13 {"image number"=-1, "image path"=path "", "position"={0.0, 0.0}}  # End Signal
                  n137 = Strip Path(path=w432) -> (stripped path=w433:path)  [unwired: 1 out]
                  n138 = Open/Create/Replace File(file path (use dialog)=w432, access (0:read/write)=enum16{"read/write", "read-only", "write-only"}."read-only") -> (refnum out=w431:refnum<file>, error out=w430:errorcluster)  [unwired: 4 in, 1 out]
                  n139 = Read from Text File(file (use dialog)=w431, count=-1, error in=w430) -> (refnum out=w428:refnum<file>, text=w434:string[], error out=w429:errorcluster)  [unwired: 1 in, 1 out]
                  n140 = Close File(refnum=w428, error in=w429) -> ()  [unwired: 2 out]
                  n141 = for {
                    N -> [w439]
                    shift-right: [w445] -> w427
                    shift-left: w436 -> [w452]
                    tunnel: w434 -> [w444] mode=indexing
                    tunnel: w433 -> [w443]
                    shift-right: [w440] -> w425
                    shift-left: w437 -> [w453]
                    n142 = local write "Loops"(w439) -> ()
                    n143 = Scan From String(format string="%d,%[^,],%f,%f", input string=w444) -> (output 1=w447:i32, output 2=w441:string, output 3=w450:dbl, output 4=w449:dbl)  [unwired: 6 in, 3 out]
                    n144 = Build Path(base path=w443, name or relative path=w441) -> (appended path=w442:path)
                    n145 = Bundle(w450, w449) -> (w448:cluster{dbl, dbl})  [unwired: 1 in]
                    n146 = Bundle(w447, "appended path"=w442, w448) -> (w446:T26)  [unwired: 1 in]
                    n147 = Enqueue Element(queue=w453, element=w446, error in (no error)=w452) -> (queue out=w440:refnum<queue>, error out=w445:errorcluster)  [unwired: 1 in, 1 out]
                  }
                  n148 = Enqueue Element(queue=w425, element=w424, error in (no error)=w427) -> (error out=w426:errorcluster)  [unwired: 1 in, 2 out]
                }
              }
              n149 = call "SmartFileName.vi"("Allow Replacement (False)"=w158, "preferred name"=w159, "preferred path"=w160) -> ("Smart Path"=w187:path)
              n150 = Open/Create/Replace File(file path (use dialog)=w187, operation (0:open)=T12."replace or create", access (0:read/write)=enum16{"read/write", "read-only", "write-only"}."write-only") -> (refnum out=w182:refnum<file>, error out=w161:errorcluster)  [unwired: 3 in, 1 out]
              n151 = Concatenate Strings("%s,%d,%.8f,%.11f,%.8f,%.8f,%.8f,%.8f,%.8f,%.8f,%.8f,%.8f,%d", "\r\n") -> (w165:string)
              n152 = while "Consumer Loop: Analyze Images" {
                shift-right: [w475] -> _
                shift-left: T11 {"Params Vector[1]"=-1.0, "Params Vector[2]"=0.0} -> [w465]
                tunnel: "Python" -> [w474]
                tunnel: w182 -> [w471]
                shift-right: [w470] -> w169
                shift-left: w161 -> [w469]
                tunnel: [w468] -> w181
                tunnel: w165 -> [w467]
                shift-right: [w466] -> w167
                shift-left: w171 -> [w477]
                i -> [w461]
                stop <- w454 stop-if-true
                n153 = local read "Loops"() -> (w462:i32)
                n154 = Dequeue Element(queue=w477) -> (queue out=w466:refnum<queue>, element=w476:T13)  [unwired: 2 in, 2 out]
                n155 = Divide(x=w461, y=w462) -> (x/y=w458:dbl)
                n156 = Format Into String(format string=" %d/%d", initial string="Progress:", w461, w462) -> (resulting string=w464:string)  [unwired: 1 in, 1 out]
                n157 = Unbundle By Name(w476) -> ("image number"=w456:i32, "position"=w473:cluster{dbl, dbl}, "image path"=w472:path)
                n158 = Multiply(x=100, y=w458) -> (x*y=w459:dbl)
                n159 = property on="Progress" class="Slide (strict)"("Value"=w459, "Caption.Text"=w464) -> ()  [unwired: 2 in, 2 out]
                n160 = Less Than 0?(x=w456) -> (x < 0?=w455:bool)
                n161 = case shown="False" w455 {
                  tunnel: [w510 w515] -> w475
                  tunnel: w474 -> [w509 _]
                  tunnel: w473 -> [w506 _]
                  tunnel: w472 -> [w493 _]
                  tunnel: w471 -> [w490 w514]
                  tunnel: [w489 w513] -> w470
                  tunnel: w469 -> [w488 w513]
                  tunnel: [w487 w514] -> w468
                  tunnel: w467 -> [w486 _]
                  tunnel: w465 -> [w480 w515]
                  tunnel: w456 -> [w479 _]
                  tunnel: [FALSE TRUE] -> w454
                  frame False {
                    # "Fit Images"
                    n162 = call "SubVI_ProcessImage.vi"("Image Path"=w493, "Path to Python.exe"=w509, "Initial Guess"=w480) -> ("Success"=w492:bool, "Params Vector"=w512:dbl[], "Errors"=w508:dbl[], "Iterations"=w494:i32)
                    n163 = Array To Cluster(array=w512) -> (cluster=w484:T27)
                    n164 = Array To Cluster(array=w508) -> (cluster=w505:T28)
                    n165 = Unbundle(w506) -> (w504:dbl, w503:dbl)
                    n166 = Unbundle(w484) -> ("Params Vector[0]"=w502:dbl, "Params Vector[1]"=w501:dbl, "Params Vector[2]"=w500:dbl)
                    n167 = Unbundle(w505) -> ("Errors[0]"=w499:dbl, "Errors[1]"=w498:dbl, "Errors[2]"=w497:dbl)
                    n168 = Unbundle(w480) -> ("Params Vector[1]"=w496:dbl, "Params Vector[2]"=w495:dbl)
                    n169 = Bundle("Success"=w492, "image number"=w479, "position"=w506, "Params Vector"=w484, "Errors"=w505, w480, "Iterations"=w494, "image path"=w493) -> (w507:T29)  [unwired: 1 in]
                    n170 = Unbundle(w484) -> ("Params Vector[1]"=w483:dbl, "Params Vector[2]"=w482:dbl)  [unwired: 1 out]
                    n171 = local read "Image Data"() -> (w511:T1)
                    n172 = Format Into String(format string=w486, w492, w479, w504, w503, w502, w501, w500, w499, w498, w497, w496, w495, w494) -> (resulting string=w491:string)  [unwired: 2 in, 1 out]
                    n173 = Build Array (concatenate)(w511, w507) -> (w485:T30)
                    n174 = Bundle("Params Vector[1]"=w483, "Params Vector[2]"=w482) -> (w481:T11)  [unwired: 1 in]
                    n175 = property on="Image Data" class="Arr (strict)"("Val(Sgnl)"=w485) -> ()  [unwired: 2 in, 2 out]
                    n176 = Write to Text File(file (use dialog)=w490, text=w491, error in=w488) -> (refnum out=w487:refnum<file>, error out=w489:errorcluster)  [unwired: 1 in, 1 out]
                    n177 = Select(t=w481, s=w492, f=w480) -> (s? t:f=w510:T11)
                  }
                  frame True {
                  }
                }
              }
              n178 = Merge Errors(w175, w169) -> (w170:errorcluster)
              n179 = Close File(refnum=w181, error in=w169) -> (error out=→"data file write error":errorcluster)  [unwired: 1 out]
              n180 = Release Queue(queue=w167, error in (no error)=w170) -> (error out=→"queue error":errorcluster)  [unwired: 1 in, 2 out]
            }
            frame "View Results" {
              n181 = property on="Image File Results Read" class="Bool (strict)"() -> ("Value"=w524:bool)  [unwired: 2 in, 2 out]
              n182 = Open/Create/Replace File(file path (use dialog)=w529, access (0:read/write)=enum16{"read/write", "read-only", "write-only"}."read-only") -> (refnum out=w528:refnum<file>, error out=w527:errorcluster)  [unwired: 4 in, 1 out]
              n183 = case shown="True" w524 {
                tunnel: w523 -> [_ w539]
                tunnel: [path "" w538] -> w522
                tunnel: [errorcluster {"status"=FALSE, "code"=0, "source"=""} ("error out") w536] -> w519
                tunnel: [string[] [] w533] -> w520
                frame False {
                }
                frame True {
                  n184 = Strip Path(path=w539) -> (stripped path=w538:path)  [unwired: 1 out]
                  n185 = Open/Create/Replace File(file path (use dialog)=w539, access (0:read/write)=enum16{"read/write", "read-only", "write-only"}."read-only") -> (refnum out=w535:refnum<file>, error out=w537:errorcluster)  [unwired: 4 in, 1 out]
                  n186 = Read from Text File(file (use dialog)=w535, count=-1, error in=w537) -> (text=w533:string[], error out=w536:errorcluster)  [unwired: 1 in, 2 out]
                }
              }
              n187 = Read from Text File(file (use dialog)=w528, count=-1, error in=w527) -> (text=w525:string[])  [unwired: 1 in, 3 out]
              n188 = for {
                N -> [w541]
                tunnel: w525 -> [w569] mode=indexing
                tunnel: "%[^,],%d,%f,%f,%f,%f,%f,%f,%f,%f,%f,%f,%d" -> [w552]
                tunnel: w524 -> [w546]
                tunnel: w522 -> [w545]
                tunnel: w520 -> [w544]
                tunnel: w519 -> [w542]
                tunnel: [w553] -> w517 mode=indexing
                i -> [w543]
                n189 = case shown="True" w546 {
                  tunnel: [path "" w575] -> w547
                  tunnel: w545 -> [_ w576]
                  tunnel: w544 -> [_ w578]
                  tunnel: w543 -> [_ w577]
                  tunnel: w542 -> [_ w574]
                  frame False {
                  }
                  frame True {
                    n190 = Index Array(array=w578, index=w577) -> (element=w571:string)
                    n191 = Scan From String(format string="%d,%[^,],", input string=w571, error in=w574) -> (output 2=w572:string)  [unwired: 4 in, 3 out]
                    n192 = Build Path(base path=w576, name or relative path=w572) -> (appended path=w575:path)
                  }
                }
                n193 = Scan From String(format string=w552, input string=w569) -> (output 1=w549:string, output 2=w558:i32, output 3=w568:dbl, output 4=w567:dbl, output 5=w566:dbl, output 6=w565:dbl, output 7=w564:dbl, output 8=w563:dbl, output 9=w562:dbl, output 10=w561:dbl, output 11=w560:dbl, output 12=w559:dbl, output 13=w551:i32)  [unwired: 15 in, 3 out]
                n194 = Bundle(w568, w567) -> (w557:cluster{dbl, dbl})  [unwired: 1 in]
                n195 = Bundle(w566, w565, w564) -> (w554:cluster{dbl, dbl, dbl})  [unwired: 1 in]
                n196 = Bundle(w563, w562, w561) -> (w556:cluster{dbl, dbl, dbl})  [unwired: 1 in]
                n197 = Bundle(w560, w559) -> (w555:cluster{dbl, dbl})  [unwired: 1 in]
                n198 = Type Cast(type=FALSE, x=w549) -> (*(type *) &x=w548:bool)
                n199 = property on="Loops" class="DigNum (strict)"("Value"=w541) -> ()  [unwired: 2 in, 2 out]
                n200 = Bundle(w548, w558, w557, w554, w556, w555, w551, "appended path"=w547) -> (w553:T31)  [unwired: 1 in]
              }
              n201 = property on="Image Data" class="Arr (strict)"("Val(Sgnl)"=w517) -> ()  [unwired: 2 in, 2 out]
            }
          }
        }
        frame #1 {
          w582 = T10."Disabled and Grayed Out" ("Disabled")
          w615 = T32 0 items=["Least Square", "Least Absolute Residual", "Bisquare"] ("method")
          w619 = T2."Results" ("Tab Control")
          # "Analyze Data/Display \"Results\" Tab"
          n202 = property on="Image Data" class="Arr (strict)"() -> ("Value"=w614:T1)  [unwired: 2 in, 2 out]
          n203 = global read "PixelToMicron.vi" "PixelToMicron"() -> (w613:dbl)
          n204 = property on="fails" class="DigNum (strict)"() -> ("Value"=w586:i32)  [unwired: 2 in, 2 out]
          n205 = property on="Loops" class="DigNum (strict)"() -> ("Value"=w585:i32)  [unwired: 2 in, 2 out]
          n206 = To Long Integer(number="percentile") -> (32bit integer=w602:i32)
          n207 = property on="Loops" class="DigNum (strict)"() -> ("Value"=w599:i32)  [unwired: 2 in, 2 out]
          n208 = Divide(x=w586, y=w585) -> (x/y=w587:dbl)
          n209 = Number To Decimal String(number=w602) -> (decimal integer string=w590:string)  [unwired: 1 in]
          n210 = Concatenate Strings(w590, "% Tolerance (microns): ") -> (w592:string)
          n211 = property on="Tab Control" class="TabCtl (strict)"("Value"=w619) -> ("Pages"=w620:refnum<vi>[])  [unwired: 2 in, 2 out]
          n212 = Greater?(x=w587, y=0.1) -> (0:→"Re-do Necessary?":bool)
          n213 = Divide(x=w613, y=1000.0) -> (x/y=w611:dbl)
          n214 = for {
            tunnel: w614 -> [w639] mode=indexing
            tunnel: w611 -> [w638]
            tunnel: [w632] -> w606 mode=indexing
            tunnel: [w631] -> w609 mode=indexing
            tunnel: [w630] -> _ mode=indexing
            tunnel: [w629] -> w583 mode=indexing
            tunnel: [w628] -> w607 mode=indexing
            n215 = Unbundle By Name(w639) -> ("success?"=w637:bool, "camera position.X"=w636:dbl, "camera position.Y"=w635:dbl, "parameters.center"=w634:dbl, "errors.center"=w633:dbl)
            n216 = case shown="False" w637 {
              selector: w637 -> [w641 w644]
              tunnel: w638 -> [_ w652]
              tunnel: w636 -> [w642 w649]
              tunnel: w635 -> [_ w650]
              tunnel: w634 -> [_ w653]
              tunnel: w633 -> [_ w646]
              tunnel: [w642 w649] -> w632
              tunnel: [w640 w648] -> w631
              tunnel: [w640 w647] -> w630
              tunnel: [w640 w643] -> w629
              tunnel: [w641 w644] -> w628
              frame False {
                w640 = 0.0
              }
              frame True {
                n217 = Square(x=w646) -> (x^2=w645:dbl)
                n218 = Multiply(x=w653, y=w652) -> (x*y=w651:dbl)
                n219 = Multiply(x=w646, y=w652) -> (x*y=w647:dbl)
                n220 = Add(x=w650, y=w651) -> (x+y=w648:dbl)
                n221 = Reciprocal(x=w645) -> (1/x=w643:dbl)
              }
            }
          }
          n222 = call <vilib>:"Linear Fit.vi"("Y"=w609, "X"=w606, "Weight"=w583, "method"=w615) -> ("Best Linear Fit"=w610:dbl[])  [unwired: 7 in, 4 out]
          n223 = Subtract(x=w609, y=w610) -> (x-y=w608:dbl[])
          n224 = for {
            tunnel: w608 -> [w624] mode=indexing
            tunnel: w607 -> [w625] mode=indexing
            tunnel: [w623] -> w595 mode=indexing
            n225 = case shown="False" w625 {
              tunnel: w624 -> [_ w627]
              tunnel: [0.0 w627] -> w623
              frame False {
              }
              frame True {
              }
            }
          }
          n226 = Multiply(x=w595, y=1000.0) -> (x*y=w594:dbl[])
          n227 = Square Root(x=w599) -> (sqrt(x)=w598:dbl)
          n228 = call <vilib>:"Std Deviation and Variance.vi"("X"=w594) -> ("standard deviation"=→"std. dev.":dbl)  [unwired: 1 in, 2 out]
          n229 = Absolute Value(x=w594) -> (abs(x)=w603:dbl[])
          n230 = To Long Integer(number=w619) -> (32bit integer=w618:i32)
          n231 = property on="Tolerance" class="DigNum (strict)"("Caption.Text"=w592) -> ("Value"=w589:dbl)  [unwired: 2 in, 2 out]
          n232 = To Long Integer(number=w598) -> (32bit integer=w597:i32)
          n233 = call-poly <vilib>:"Percentiles.vi"("p"="percentile", "x array"=w603) -> ("percentile"=w588:dbl)  [unwired: 8 in, 1 out]
          n234 = Concatenate Strings(w590, "% Confidence Interval (microns): ") -> (w601:string)
          n235 = Index Array(array=w620, index=w618) -> (element=w622:refnum<vi>)
          n236 = call <vilib>:"Histogram.vi"("intervals"=w597, "X"=w595) -> ("Histogram Graph"=→"Histogram of Final Fit Residuals":T9)  [unwired: 6 in, 3 out]
          n237 = property on="Progress" class="Slide (strict)"("Value"=u8 100 ("Progress"), "Caption.Text"="Progress: complete") -> ()  [unwired: 2 in, 2 out]
          n238 = property on="confidence" class="DigNum (strict)"("Value"=w588, "Caption.Text"=w601) -> ()  [unwired: 2 in, 2 out]
          n239 = Greater?(x=w588, y=w589) -> (0:→"outside tolerance":bool)
          n240 = Bundle(w606, w595) -> (→"Adjusted Graph of Final Fit":cluster{dbl[], dbl[]})  [unwired: 1 in]
          n241 = property class="Page"(reference=w622, "PageVis"=TRUE ("Page Visible")) -> ()  [unwired: 1 in, 2 out]
          n242 = property on="abort" class="Bool"("DisabledEnum"=w582) -> ()  [unwired: 2 in, 2 out]
          n243 = property on="pause" class="Bool (strict)"("DisabledEnum"=w582) -> ()  [unwired: 2 in, 2 out]
        }
      }
      n244 = local read "Mode"() -> (w63:enum16{"Run Calibration", "View Results"})
      n245 = global read "PixelToMicron.vi" "PixelToMicron"() -> (w84:dbl)
      n246 = Equal To 0?(x=w63) -> (x = 0?=w61:bool)
      n247 = Not Or(1:w60, 2:w61) -> (0:w62:bool)
      n248 = Select(t=T10."Disabled and Grayed Out" ("Disabled"), s=w62, f=T10."Enabled" ("Disabled")) -> (s? t:f=w65:T10)
      n249 = Divide(x=w84, y=1000.0) -> (x/y=w82:dbl)
      n250 = while "Listener Loop: Load Lists in \"Data\" Tab" {
        tunnel: w82 -> [w90]
        stop <- w89 stop-if-true
        n251 = event shown="[1] \"Image Data\": Value Change" {
          selector: _ -> [_ _ _]
          dyn-events: _ -> [_ _ _]
          timeout: -1 -> [_ _ _]
          tunnel: w90 -> [_ w105 _]
          tunnel: [TRUE FALSE w138] -> w89
          event Timeout {
            n252 = event-data() -> ()  [unwired: 1 in, 3 out]
          }
          event "Image Data": Value Change {
            n253 = event-data() -> ("NewVal"=w104:T1, "OldVal"=w103:T1)  [unwired: 1 in]
            n254 = Array Size(array=w103) -> (size(s)=w102:i32)
            n255 = Array Subset(array=w104, index=w102) -> (w101:T1)  [unwired: 1 in]
            n256 = for {
              tunnel: w105 -> [w123]
              tunnel: w101 -> [w110] mode=indexing
              tunnel: [w108] -> w95 mode=indexing
              tunnel: [w107] -> w94 mode=indexing
              tunnel: ",%d,%.8f,%.11f,%.11f,%d" -> [w106]
              n257 = Unbundle By Name(w110) -> ("image number"=w122:i32, "camera position.X"=w121:dbl, "camera position.Y"=w124:dbl, "parameters.center"=w126:dbl, "errors.center"=w127:dbl, "iterations"=w118:i32, "success?"=w109:bool)
              n258 = Multiply(x=w123, y=w126) -> (x*y=w125:dbl)
              n259 = Multiply(x=w123, y=w127) -> (x*y=w119:dbl)
              n260 = Add(x=w124, y=w125) -> (x+y=w120:dbl)
              n261 = Format Into String(format string=w106, w122, w121, w120, w119, w118) -> (resulting string=w117:string)  [unwired: 2 in, 1 out]
              n262 = Spreadsheet String To Array(delimiter (Tab)=",", format string="%s", spreadsheet string=w117, array type (2D Dbl)="") -> (array=w112:string[][])
              n263 = Select(t=1, s=w109, f=2) -> (s? t:f=w107:i32)
              n264 = Index Array(array=w112) -> (element=w108:string[])  [unwired: 2 in]
              n265 = case shown="False" w109 {
                tunnel: w108 -> [w136 _]
                frame False {
                  n266 = property on="List of Failed Fits" class="MCListbox (strict)"() -> (error out=w130:errorcluster, "ItemNames"=w131:string[][])  [unwired: 2 in, 1 out]
                  n267 = Index Array(array=w136, index #1=1) -> (element #1=w135:string, element #2=w134:string)  [unwired: 1 in]
                  n268 = Build Array(w135, w134) -> (w132:string[])
                  n269 = property on="fails" class="DigNum (strict)"() -> ("Value"=w129:i32)  [unwired: 2 in, 2 out]
                  n270 = Build Array (concatenate)(w131, w132) -> (w133:string[][])
                  n271 = Increment(x=w129) -> (x+1=w128:i32)
                  n272 = property on="List of Failed Fits" class="MCListbox (strict)"(error in=w130, "ItemNames"=w133) -> ()  [unwired: 1 in, 2 out]
                  n273 = property on="fails" class="DigNum (strict)"("Value"=w128) -> ()  [unwired: 2 in, 2 out]
                }
                frame True {
                }
              }
            }
            n274 = property on="List of All Fits" class="MCListbox (strict)"() -> (error out=w98:errorcluster, "ItemNames"=w99:string[][], "ItemSyms"=w97:i32[])  [unwired: 2 in, 1 out]
            n275 = Build Array (concatenate)(w99, w95) -> (w93:string[][])
            n276 = Build Array (concatenate)(w97, w94) -> (w96:i32[])
            n277 = property on="List of All Fits" class="MCListbox (strict)"(error in=w98, "ItemNames"=w93, "ItemSyms"=w96) -> ()  [unwired: 1 in, 2 out]
          }
          event "Quit": Value Change {
            n278 = event-data() -> ("NewVal"=w138:bool)  [unwired: 1 in]
          }
        }
      }
      n279 = property on="Image" class="ImageControl"("DisabledEnum"=w65) -> ()  [unwired: 2 in, 2 out]
      n280 = property on="Graph of Fit" class="XYGraph (strict)"("DisabledEnum"=w65) -> ()  [unwired: 2 in, 2 out]
      n281 = property on="Tab Control" class="TabCtl (strict)"("Value"=w81) -> ("Pages"=w85:refnum<vi>[])  [unwired: 2 in, 2 out]
      n282 = To Long Integer(number=w81) -> (32bit integer=w80:i32)
      n283 = Index Array(array=w85, index=w80) -> (element=w87:refnum<vi>)
      n284 = property class="Page"(reference=w87, "PageVis"=TRUE ("Page Visible")) -> ()  [unwired: 1 in, 2 out]
      n285 = property on="View Results" class="Bool"("DisabledEnum"=w59) -> ()  [unwired: 2 in, 2 out]
      n286 = property on="Run Calibration" class="Bool"("DisabledEnum"=w59) -> ()  [unwired: 2 in, 2 out]
      n287 = property on="List of All Fits" class="MCListbox (strict)"("ItemNames"=string[][] [] ("Item Names"), "Symbols Vis"=TRUE ("Visible Items:Symbols Visible")) -> ()  [unwired: 2 in, 2 out]
      n288 = property on="List of Failed Fits" class="MCListbox (strict)"("ItemNames"=string[][] [] ("Item Names")) -> ()  [unwired: 2 in, 2 out]
      n289 = while "Listener Loop: Display \"Data\" Tab" {
        shift-right: [w657] -> _
        shift-left: errorcluster {"status"=FALSE, "code"=0, "source"=""} ("error out") -> [w656]
        shift-right: [w655] -> _
        shift-left: _ -> [w654]
        stop <- w659 stop-if-true
        n290 = event shown="[2] \"List of All Fits\": Value Change" {
          selector: _ -> [_ _ _ _ _]
          dyn-events: _ -> [_ _ _ _ _]
          timeout: -1 -> [_ _ _ _ _]
          tunnel: [TRUE FALSE w674 FALSE w758] -> w659
          tunnel: [w661 w666 w678 w754 w757] -> w657
          tunnel: w656 -> [w661 w666 w673 w754 w757]
          tunnel: [w660 w663 w672 w744 w756] -> w655
          tunnel: w654 -> [w660 w663 w671 w744 w756]
          event Timeout {
            n291 = event-data() -> ()  [unwired: 1 in, 3 out]
          }
          event "List of Failed Fits": Value Change {
            n292 = event-data() -> ("NewVal"=w665:i32)  [unwired: 1 in]
            n293 = property on="List of Failed Fits" class="MCListbox (strict)"() -> ("ItemNames"=w669:string[][])  [unwired: 2 in, 2 out]
            n294 = Index Array(array=w669, index (row)=w665, index (col)=0) -> (element=w668:string)
            n295 = Decimal String To Number(string=w668) -> (number=w664:i32)  [unwired: 2 in, 1 out]
            n296 = property on="List of All Fits" class="MCListbox (strict)"("Val(Sgnl)"=w664) -> ()  [unwired: 2 in, 2 out]
          }
          event "List of All Fits": Value Change {
            n297 = event-data() -> ("OldVal"=w677:i32, "NewVal"=w675:i32)  [unwired: 1 in]
            n298 = property on="Image Data" class="Arr (strict)"() -> ("Value"=w679:T1)  [unwired: 2 in, 2 out]
            n299 = Not Equal?(x=w677, y=w675) -> (x != y?=w676:bool)
            n300 = case shown="True" w676 {
              tunnel: w679 -> [_ w737]
              tunnel: w673 -> [w682 w685]
              tunnel: [w682 w692] -> w678
              tunnel: w675 -> [_ w723]
              tunnel: [FALSE FALSE] -> w674
              tunnel: [w680 w686] -> w672
              tunnel: w671 -> [w680 w684]
              frame False {
              }
              frame True {
                w730 = T21 0 items=["Grayscale (U8)", "Grayscale (I16)", "Grayscale (SGL)", "Complex (CSG)", "RGB (U32)", "HSL (U32)", "RGB (U64)", "Grayscale (U16)"] ("Image Type")
                n301 = call "IMAQ Dispose"("Image"=w684, "error in (no error)"=w685) -> ()  [unwired: 4 in, 1 out]
                n302 = Index Array(array=w737, index=w723) -> (element=w736:T33)
                n303 = property on="Wire Diameter" class="DigNum (strict)"() -> ("Value"=w712:dbl)  [unwired: 2 in, 2 out]
                n304 = global read "PixelToMicron.vi" "PixelToMicron"() -> (w713:dbl)
                n305 = Unbundle By Name(w736) -> ("Initial Guess"=w734:cluster{"center":dbl, "reflectivity":dbl}, "parameters"=w714:T34, "errors"=w735:T34, "iterations"=w732:i32, "success?"=w731:bool, "image path"=w725:path, "image number"=w721:i32)
                n306 = Format Into String(format string="%d", initial string="Image #", w721) -> (resulting string=w716:string)  [unwired: 1 in, 1 out]
                n307 = Divide(x=w712, y=w713) -> (x/y=w701:dbl)
                n308 = Multiply(x=1.5, y=w701) -> (x*y=w708:dbl)
                n309 = Unbundle By Name(w714) -> ("center"=w710:dbl)
                n310 = Concatenate Strings("Graph of Fit for " ("string"), w716) -> (w718:string)
                n311 = Scale By Power Of 2(n=i16 -1, x=w701) -> (x*2^n=w699:dbl)
                n312 = Cluster To Array(cluster=w714) -> (array=w700:dbl[])
                n313 = Cluster To Array(cluster=w735) -> (array=w733:dbl[])
                n314 = Scale By Power Of 2(n=i16 1, x=w708) -> (x*2^n=w707:dbl)
                n315 = property on="Image" class="ImageControl"("Caption.Text"=w716) -> ()  [unwired: 2 in, 2 out]
                n316 = property on="Graph of Fit" class="XYGraph (strict)"("Caption.Text"=w718) -> ()  [unwired: 2 in, 2 out]
                n317 = Subtract(x=w710, y=w708) -> (x-y=w706:dbl)
                n318 = Bundle("Initial Guess"=w734, "parameters"=w700, "errors"=w733, "iterations"=w732, "success?"=w731) -> (→"Fit Info":T35)  [unwired: 1 in]
                n319 = To Long Integer(number=w706) -> (32bit integer=w704:i32)
                n320 = To Long Integer(number=w707) -> (32bit integer=w705:i32)
                n321 = for {
                  N: w705 -> [_]
                  tunnel: w704 -> [w742]
                  tunnel: [w741] -> w703 mode=indexing
                  i -> [w743]
                  n322 = Add(x=w742, y=w743) -> (x+y=w741:i32)
                }
                n323 = Strip Path(path=w725) -> (name=w726:string)  [unwired: 1 out]
                n324 = Search/Split String(string=w726, search string/char (-)=".") -> (substring before match=w728:string)  [unwired: 1 in, 2 out]
                n325 = To Double Precision Float(number=w703) -> (double precision float=w690:dbl[])
                n326 = Build Array (concatenate)(w700, w699) -> (w689:dbl[])
                n327 = call "IMAQ Create"("Image Name"=w728, "Image Type"=w730, "error in (no error)"=w685) -> ("New Image"=w727:T7, "error out"=w724:errorcluster)  [unwired: 2 in]
                n328 = for {
                  tunnel: [w740] -> w691 mode=indexing
                  tunnel: w690 -> [w739] mode=indexing
                  tunnel: w689 -> [w738]
                  n329 = call "JoelReflectivityModel.vi"("Parameters"=w738, "x"=w739) -> ("y"=w740:dbl)  [unwired: 8 in, 1 out]
                }
                n330 = call "IMAQ ReadFile"("File Path"=w725, "error in (no error)"=w724, "Image"=w727) -> ("error out"=w715:errorcluster, "Image Out"=w686:T7)  [unwired: 4 in, 3 out]
                "Image" <- w686
                n331 = call "GetImageData.vi"("error in (no error)"=w715, "Image"=w686) -> ("error out"=w692:errorcluster, "Array"=w688:dbl[])  [unwired: 7 in]
                n332 = call "SimpleVariance.vi"("X"=w688) -> ("variance"=w687:dbl[])  [unwired: 1 in, 1 out]
                n333 = Array Subset(array=w687, index=w704, length=w705) -> (w697:dbl[])
                n334 = Bundle(w690, w697) -> (w695:cluster{dbl[], dbl[]})  [unwired: 1 in]
                n335 = Select(t=dbl[] [], s=w692, f=w691) -> (s? t:f=w693:dbl[])
                n336 = Bundle(w690, "t"=w693) -> (w696:cluster{dbl[], "t":dbl[]})  [unwired: 1 in]
                n337 = Build Array(w695, w696) -> (w698:cluster{dbl[], "t":dbl[]}[])
                n338 = property on="Graph of Fit" class="XYGraph (strict)"("Value"=w698) -> ()  [unwired: 2 in, 2 out]
              }
            }
            "Image Display Error" <- w673
          }
          event "Image Data": Value Change {
            n339 = event-data() -> ("OldVal"=w750:T1, "NewVal"=w753:T1)  [unwired: 1 in]
            n340 = property on="List of All Fits" class="MCListbox (strict)"() -> ("Value"=w751:i32)  [unwired: 2 in, 2 out]
            n341 = Increment(x=w751) -> (x+1=w746:i32)
            n342 = Array Size(array=w750) -> (size(s)=w749:i32)
            n343 = Equal?(x=w746, y=w749) -> (x = y?=w748:bool)
            n344 = Array Size(array=w753) -> (size(s)=w747:i32)
            n345 = Decrement(x=w747) -> (x-1=w745:i32)
            n346 = case shown="True" w748 {
              tunnel: w745 -> [_ w755]
              frame False {
              }
              frame True {
                n347 = property on="List of All Fits" class="MCListbox (strict)"("Val(Sgnl)"=w755) -> ()  [unwired: 2 in, 2 out]
              }
            }
          }
          event "Quit": Value Change {
            n348 = event-data() -> ("NewVal"=w758:bool)  [unwired: 1 in]
          }
        }
      }
    }
  }
  n349 = while "Show/Hide Troubleshooting Tab" {
    stop <- w760 stop-if-true
    n350 = event shown="[2] \"error tab\": Value Change" {
      selector: _ -> [_ _ _]
      dyn-events: _ -> [_ _ _]
      timeout: -1 -> [_ _ _]
      tunnel: [TRUE ("NewVal") w762 FALSE ("NewVal")] -> w760
      event Timeout {
        n351 = event-data() -> ()  [unwired: 1 in, 1 out]
      }
      event "Quit": Value Change {
        n352 = event-data() -> ("NewVal"=w762:bool)  [unwired: 1 in]
      }
      event "error tab": Value Change {
        n353 = event-data() -> ("NewVal"=w765:bool)  [unwired: 1 in]
        n354 = property on="Tab Control" class="TabCtl (strict)"() -> ("Pages"=w767:refnum<vi>[])  [unwired: 2 in, 2 out]
        n355 = Index Array(array=w767, index=3) -> (element=w766:refnum<vi>)
        n356 = property class="Page"(reference=w766, "PageVis"=w765) -> ()  [unwired: 1 in, 2 out]
      }
    }
  }
